vi "Update.vi"(8 "error in (no error)":errorcluster, 10 "Message in":refnum<class "UpdateMessage.lvclass">, 11 "Waveform in":refnum<class "Waveform.lvclass">) -> (0 "error out":errorcluster, 3 "Waveform out":refnum<class "Waveform.lvclass">)   [LabVIEW 2012, in "Waveform.lvclass"]
doc: "The update method processes the command 'update'. \n\nThe command 'update' is used for receiving new values to be set to the private data of the class. This could be seen as a public set method for setting new parameters to the private class data."
uses:
  Waveform.lvclass
  <vilib>/Distrio/Murmex/UpdateMessage/UpdateMessage.lvclass
  PC_wavelength.ctl
  Waveform.lvclass/Waveform.ctl
  <vilib>/Distrio/Murmex/Murmex/Murmex.lvclass
panel:
  # "This method is called when the UPDATE\ntrigger is sent. \n\nOverride this method when your component needs to\nrespond to this trigger. \n\nCall parent for proper implementation"
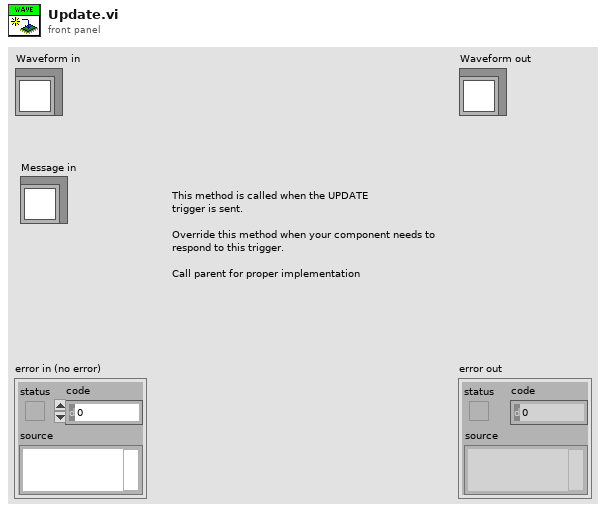
[diagram p1: front panel]
types:
  T1 = typedef "PC_wavelength.ctl" = dbl
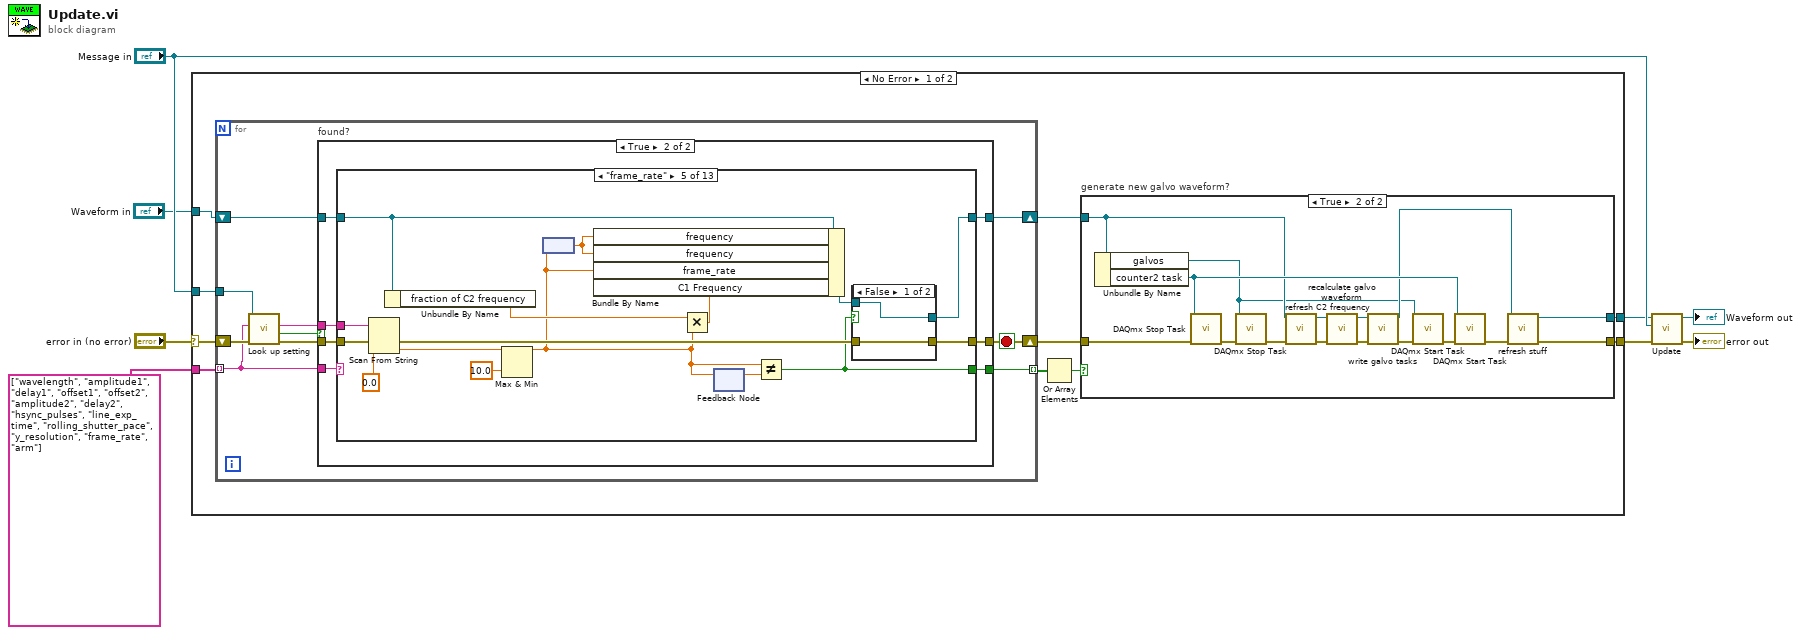
[diagram p0: block diagram]
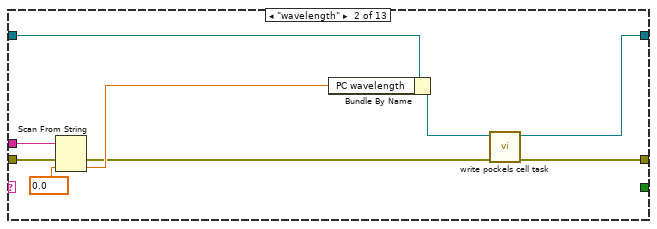
[diagram p5: hidden frame]
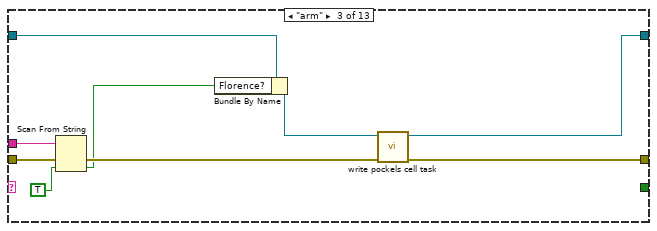
[diagram p6: hidden frame]
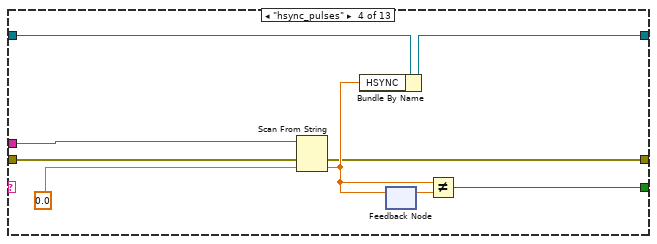
[diagram p7: hidden frame]
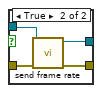
[diagram p8: hidden frame]
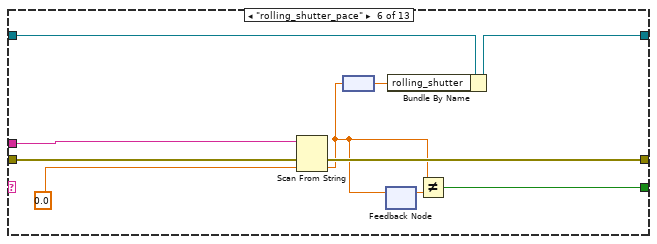
[diagram p9: hidden frame]
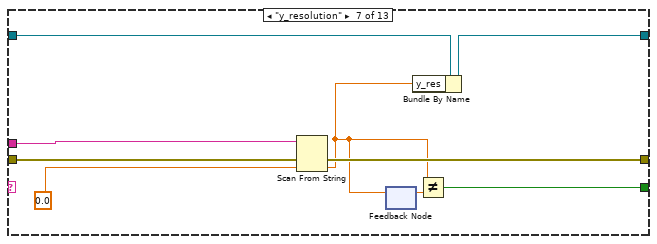
[diagram p10: hidden frame]
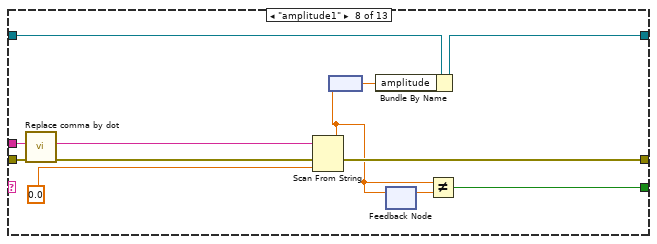
[diagram p11: hidden frame]
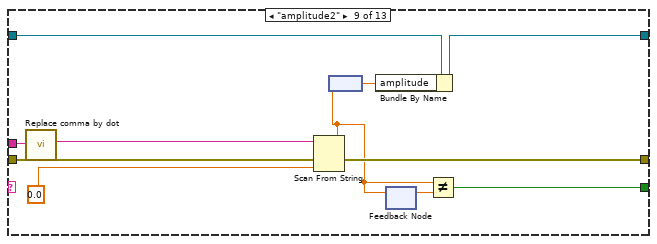
[diagram p12: hidden frame]
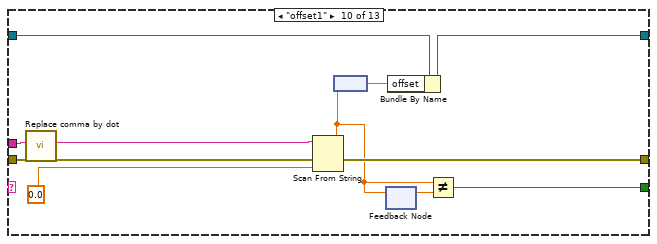
[diagram p13: hidden frame]
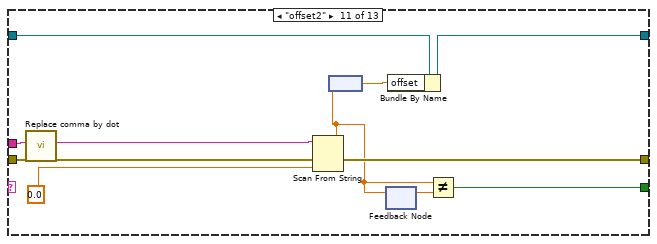
[diagram p14: hidden frame]
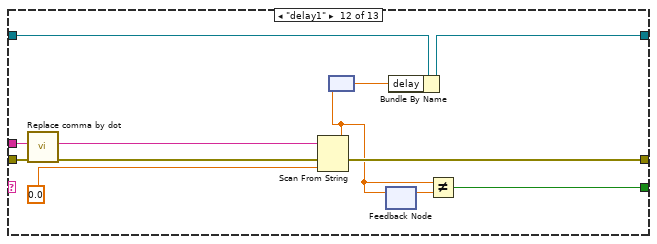
[diagram p15: hidden frame]
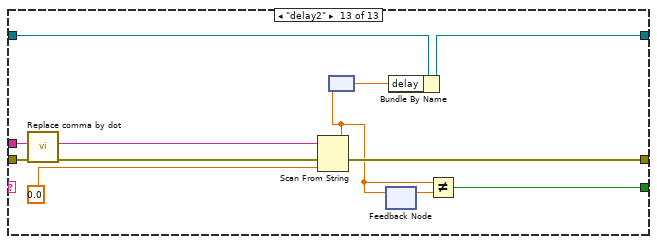
[diagram p16: hidden frame]
diagram:
  n1 = case shown="No Error" "error in (no error)" {
    selector: "error in (no error)" -> [w18 w193]
    tunnel: "Message in" -> [w17 _]
    tunnel: "Waveform in" -> [w16 w194]
    tunnel: string[] ["wavelength", "amplitude1", "delay1", "offset1", "offset2", "amplitude2", "delay2", "hsync_pulses", "line_exp_time", "rolling_shutter_pace", "y_resolution", "frame_rate", "arm"] ("key chains") -> [w15 _]
    tunnel: [w11 w193] -> w3
    tunnel: [w10 w194] -> w2
    frame No Error {
      n2 = for {
        shift-right: [w39] -> w12
        shift-left: w18 -> [w46]
        tunnel: w17 -> [w45]
        shift-right: [w40] -> w9
        shift-left: w16 -> [w44]
        tunnel: w15 -> [w37] mode=indexing
        tunnel: [w38] -> w14 mode=indexing
        stop <- w39 stop-if-true
        n3 = call <vilib>:"Look up setting.vi"("error in (no error)"=w46, "tag name"=w37, "UpdateMessage in"=w45) -> ("error out"=w43:errorcluster, "found?"=w42:bool, "value"=w41:string)  [unwired: 5 in, 1 out]
        n4 = case "found?" shown="True" w42 {
          selector: w42 -> [w47 _]
          tunnel: w44 -> [w49 w55]
          tunnel: w43 -> [w48 w56]
          tunnel: w41 -> [_ w51]
          tunnel: w37 -> [_ w53]
          tunnel: [w49 w54] -> w40
          tunnel: [w48 w52] -> w39
          tunnel: [w47 w50] -> w38
          frame False {
          }
          frame True {
            n5 = case shown="\"frame_rate\"" w53 {
              tunnel: w56 -> [w57 w67 w76 w85 w101 w117 w126 w137 w148 w159 w170 w181 w192]
              tunnel: w55 -> [w58 w66 w75 w84 w95 w116 w125 w136 w147 w158 w169 w180 w191]
              tunnel: [w58 w61 w72 w78 w90 w115 w124 w135 w146 w157 w168 w179 w190] -> w54
              tunnel: [w57 w62 w73 w77 w92 w114 w123 w134 w145 w156 w167 w178 w189] -> w52
              tunnel: w51 -> [_ w64 w74 w83 w100 w113 w122 w128 w139 w150 w161 w172 w183]
              tunnel: [_ _ _ w80 w89 w111 w120 w132 w143 w154 w165 w176 w187] -> w50
              frame Default {
              }
              frame "wavelength" {
                w65 = T1 0.0 items=["405nm"=0.24, "445nm"=0.26, "491nm"=0.29, "515nm"=0.3, "561nm"=0.33] ("settings.Pockels Cell.PC wavelength")
                n6 = Scan From String(input string=w64, error in=w67, default 1=w65) -> (error out=w59:errorcluster, output 1=w63:T1)  [unwired: 2 in, 2 out]
                n7 = Bundle By Name(cluster=w66, "PC wavelength"=w63) -> (w60:refnum<class "Waveform.lvclass">)
                n8 = call-dynamic "write pockels cell task.vi"("error in (no error)"=w59, "Waveform in"=w60) -> ("error out"=w62:errorcluster, "Waveform out"=w61:refnum<class "Waveform.lvclass">)  [unwired: 8 in]
              }
              frame "arm" {
                n9 = Scan From String(input string=w74, error in=w76, default 1=TRUE) -> (error out=w70:errorcluster, output 1=w68:bool)  [unwired: 2 in, 2 out]
                n10 = Bundle By Name(cluster=w75, "Florence?"=w68) -> (w71:refnum<class "Waveform.lvclass">)
                n11 = call-dynamic "write pockels cell task.vi"("error in (no error)"=w70, "Waveform in"=w71) -> ("error out"=w73:errorcluster, "Waveform out"=w72:refnum<class "Waveform.lvclass">)  [unwired: 8 in]
              }
              frame "hsync_pulses" {
                n12 = Scan From String(input string=w83, error in=w85, default 1=0.0) -> (error out=w77:errorcluster, output 1=w81:dbl)  [unwired: 2 in, 2 out]
                n13 = Bundle By Name(cluster=w84, "HSYNC"=w81) -> (w78:refnum<class "Waveform.lvclass">)
                n14 = feedback #1() -> (w82:dbl)  [unwired: 1 in]
                n15 = feedback-in #1(w81) -> ()
                n16 = Not Equal?(x=w81, y=w82) -> (x != y?=w80:bool)
              }
              frame "frame_rate" {
                n17 = Scan From String(input string=w100, error in=w101, default 1=0.0) -> (error out=w93:errorcluster, output 1=w87:dbl)  [unwired: 2 in, 2 out]
                n18 = Unbundle By Name(w95) -> ("fraction of C2 frequency"=w94:dbl)
                n19 = Max & Min(x=w87, y=10.0) -> (max(x,y)=w86:dbl)  [unwired: 1 out]
                n20 = node(w86) -> (w96:dbl[unit])
                n21 = Multiply(x=w94, y=w86) -> (x*y=w97:dbl)
                n22 = Bundle By Name(cluster=w95, "frequency"=w96, "frequency"=w96, "frame_rate"=w86, "C1 Frequency"=w97) -> (w91:refnum<class "Waveform.lvclass">)
                n23 = feedback #2() -> (w99:dbl)  [unwired: 1 in]
                n24 = feedback-in #2(w86) -> ()
                n25 = Not Equal?(x=w86, y=w99) -> (x != y?=w89:bool)
                n26 = case shown="False" w89 {
                  tunnel: w93 -> [w102 w107]
                  tunnel: [w102 w106] -> w92
                  tunnel: w91 -> [w103 w105]
                  tunnel: [w103 w104] -> w90
                  frame False {
                  }
                  frame True {
                    n27 = call-dynamic "send frame rate.vi"("error in (no error)"=w107, "Waveform in"=w105) -> ("error out"=w106:errorcluster, "Waveform out"=w104:refnum<class "Waveform.lvclass">)  [unwired: 8 in]
                  }
                }
              }
              frame "rolling_shutter_pace" {
                n28 = Scan From String(input string=w113, error in=w117, default 1=0.0) -> (error out=w114:errorcluster, output 1=w108:dbl)  [unwired: 2 in, 2 out]
                n29 = node(w108) -> (w109:dbl[unit])
                n30 = feedback #3() -> (w112:dbl)  [unwired: 1 in]
                n31 = feedback-in #3(w108) -> ()
                n32 = Bundle By Name(cluster=w116, "rolling_shutter"=w109) -> (w115:refnum<class "Waveform.lvclass">)
                n33 = Not Equal?(x=w108, y=w112) -> (x != y?=w111:bool)
              }
              frame "y_resolution" {
                n34 = Scan From String(input string=w122, error in=w126, default 1=0.0) -> (error out=w123:errorcluster, output 1=w118:dbl)  [unwired: 2 in, 2 out]
                n35 = feedback #4() -> (w121:dbl)  [unwired: 1 in]
                n36 = feedback-in #4(w118) -> ()
                n37 = Bundle By Name(cluster=w125, "y_res"=w118) -> (w124:refnum<class "Waveform.lvclass">)
                n38 = Not Equal?(x=w118, y=w121) -> (x != y?=w120:bool)
              }
              frame "amplitude1" {
                n39 = call <vilib>:"Replace comma by dot.vi"("input string"=w128) -> ("result string"=w127:string)  [unwired: 10 in]
                n40 = Scan From String(input string=w127, error in=w137, default 1=0.0) -> (error out=w134:errorcluster, output 1=w130:dbl)  [unwired: 2 in, 2 out]
                n41 = node(w130) -> (w131:dbl[unit])
                n42 = Bundle By Name(cluster=w136, "amplitude"=w131) -> (w135:refnum<class "Waveform.lvclass">)
                n43 = feedback #5() -> (w133:dbl)  [unwired: 1 in]
                n44 = feedback-in #5(w130) -> ()
                n45 = Not Equal?(x=w130, y=w133) -> (x != y?=w132:bool)
              }
              frame "amplitude2" {
                n46 = call <vilib>:"Replace comma by dot.vi"("input string"=w139) -> ("result string"=w138:string)  [unwired: 10 in]
                n47 = Scan From String(input string=w138, error in=w148, default 1=0.0) -> (error out=w145:errorcluster, output 1=w141:dbl)  [unwired: 2 in, 2 out]
                n48 = node(w141) -> (w142:dbl[unit])
                n49 = Bundle By Name(cluster=w147, "amplitude"=w142) -> (w146:refnum<class "Waveform.lvclass">)
                n50 = feedback #6() -> (w144:dbl)  [unwired: 1 in]
                n51 = feedback-in #6(w141) -> ()
                n52 = Not Equal?(x=w141, y=w144) -> (x != y?=w143:bool)
              }
              frame "offset1" {
                n53 = call <vilib>:"Replace comma by dot.vi"("input string"=w150) -> ("result string"=w149:string)  [unwired: 10 in]
                n54 = Scan From String(input string=w149, error in=w159, default 1=0.0) -> (error out=w156:errorcluster, output 1=w152:dbl)  [unwired: 2 in, 2 out]
                n55 = node(w152) -> (w153:dbl[unit])
                n56 = feedback #7() -> (w155:dbl)  [unwired: 1 in]
                n57 = feedback-in #7(w152) -> ()
                n58 = Bundle By Name(cluster=w158, "offset"=w153) -> (w157:refnum<class "Waveform.lvclass">)
                n59 = Not Equal?(x=w152, y=w155) -> (x != y?=w154:bool)
              }
              frame "offset2" {
                n60 = call <vilib>:"Replace comma by dot.vi"("input string"=w161) -> ("result string"=w160:string)  [unwired: 10 in]
                n61 = Scan From String(input string=w160, error in=w170, default 1=0.0) -> (error out=w167:errorcluster, output 1=w163:dbl)  [unwired: 2 in, 2 out]
                n62 = node(w163) -> (w164:dbl[unit])
                n63 = feedback #8() -> (w166:dbl)  [unwired: 1 in]
                n64 = feedback-in #8(w163) -> ()
                n65 = Bundle By Name(cluster=w169, "offset"=w164) -> (w168:refnum<class "Waveform.lvclass">)
                n66 = Not Equal?(x=w163, y=w166) -> (x != y?=w165:bool)
              }
              frame "delay1" {
                n67 = call <vilib>:"Replace comma by dot.vi"("input string"=w172) -> ("result string"=w171:string)  [unwired: 10 in]
                n68 = Scan From String(input string=w171, error in=w181, default 1=0.0) -> (error out=w178:errorcluster, output 1=w174:dbl)  [unwired: 2 in, 2 out]
                n69 = node(w174) -> (w175:dbl[unit])
                n70 = feedback #9() -> (w177:dbl)  [unwired: 1 in]
                n71 = feedback-in #9(w174) -> ()
                n72 = Bundle By Name(cluster=w180, "delay"=w175) -> (w179:refnum<class "Waveform.lvclass">)
                n73 = Not Equal?(x=w174, y=w177) -> (x != y?=w176:bool)
              }
              frame "delay2" {
                n74 = call <vilib>:"Replace comma by dot.vi"("input string"=w183) -> ("result string"=w182:string)  [unwired: 10 in]
                n75 = Scan From String(input string=w182, error in=w192, default 1=0.0) -> (error out=w189:errorcluster, output 1=w185:dbl)  [unwired: 2 in, 2 out]
                n76 = node(w185) -> (w186:dbl[unit])
                n77 = feedback #10() -> (w188:dbl)  [unwired: 1 in]
                n78 = feedback-in #10(w185) -> ()
                n79 = Bundle By Name(cluster=w191, "delay"=w186) -> (w190:refnum<class "Waveform.lvclass">)
                n80 = Not Equal?(x=w185, y=w188) -> (x != y?=w187:bool)
              }
            }
          }
        }
      }
      n81 = Or Array Elements(Boolean array=w14) -> (logical OR=w13:bool)
      n82 = case "generate new galvo waveform?" shown="True" w13 {
        tunnel: w12 -> [w19 w34]
        tunnel: [w19 w28] -> w11
        tunnel: [w20 w29] -> w10
        tunnel: w9 -> [w20 w25]
        frame False {
        }
        frame True {
          n83 = Unbundle By Name(w25) -> ("galvos"=w21:refnum<k21>, "counter2 task"=w33:refnum<k21>)
          n84 = call <vilib>:"DAQmx Stop Task.vi"("task/channels in"=w33, "error in"=w34) -> ("error out"=w27:errorcluster)  [unwired: 12 in, 1 out]
          n85 = call <vilib>:"DAQmx Stop Task.vi"("task/channels in"=w21, "error in"=w27) -> ("error out"=w26:errorcluster)  [unwired: 12 in, 1 out]
          n86 = call-dynamic "refresh C2 frequency.vi"("error in (no error)"=w26, "Waveform in"=w25) -> ("error out"=w32:errorcluster, "Waveform out"=w31:refnum<class "Waveform.lvclass">)  [unwired: 8 in]
          n87 = call-dynamic "recalculate galvo waveform.vi"("error in (no error)"=w32, "Waveform in"=w31) -> ("error out"=w36:errorcluster, "Waveform out"=w35:refnum<class "Waveform.lvclass">)  [unwired: 8 in]
          n88 = call-dynamic "write galvo tasks.vi"("error in (no error)"=w36, "Waveform in"=w35) -> ("error out"=w23:errorcluster, "Waveform out"=w22:refnum<class "Waveform.lvclass">)  [unwired: 8 in]
          n89 = call <vilib>:"DAQmx Start Task.vi"("task/channels in"=w21, "error in"=w23) -> ("error out"=w24:errorcluster)  [unwired: 12 in, 1 out]
          n90 = call <vilib>:"DAQmx Start Task.vi"("task/channels in"=w33, "error in"=w24) -> ("error out"=w30:errorcluster)  [unwired: 12 in, 1 out]
          n91 = call-dynamic "refresh stuff.vi"("error in (no error)"=w30, "Waveform in"=w22) -> ("error out"=w28:errorcluster, "Waveform out"=w29:refnum<class "Waveform.lvclass">)  [unwired: 8 in]
        }
      }
    }
    frame Error {
    }
  }
  n92 = call-parent "Update.vi"("error in (no error)"=w3, "Message in"="Message in", "Murmex in"=w2) -> ("error out"=→"error out":errorcluster, "Murmex out"=→"Waveform out":refnum<class "Waveform.lvclass">)  [unwired: 7 in]
